vi "XYZStage-Request motor move all axes command.vi"(6 "Wait for acknowledge?":bool, 9 "Motor Z":sgl, 10 "Motor Y":sgl, 11 "Motor X":sgl) -> (1 "Timed out while waiting for acknowledgement":bool, 2 "Acknowledgement message":string)   [LabVIEW 2013]
doc: "Sends a request to the XYZ Stage driver to move the motor to the specified position on the Z axis."
uses:
  Typedefs/XYZ stage states.ctl
  Typedefs/XYZ stage data.ctl
  Typedefs/XYZ channel ring.ctl
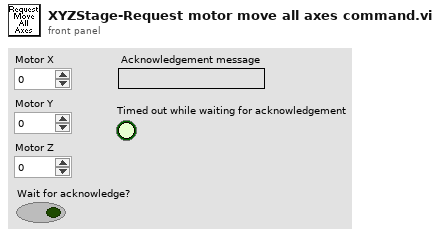
[diagram p1: front panel]
types:
  T1 = typedef "XYZ channel ring.ctl" = string
  T2 = typedef "XYZ stage data.ctl" = cluster{"Command":T3, "Channel":T1, "X":sgl, "Y":sgl, "Z":sgl, "Speed":i32, "Zero":bool, "Use acknowledgement?":bool}
  T3 = typedef "XYZ stage states.ctl" = enum16{"Dequeue", "Initialize", "Read Position", "Read Speed Setting", "Move", "Set Max Speed", "Reset Axis", "Stop all movement"}
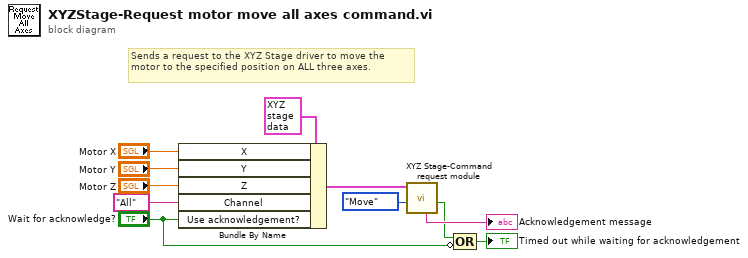
[diagram p0: block diagram]
diagram:
  # "Sends a request to the XYZ Stage driver to move the motor to the specified position on ALL three axes."
  n1 = Bundle By Name(cluster=T2 {"Command"=enum."Initialize", "Channel"="", "X"=0.0, "Y"=0.0, "Z"=0.0, "Speed"=0, "Zero"=TRUE, "Use acknowledgement?"=FALSE} ("XYZ Stage data to queue"), "X"="Motor X", "Y"="Motor Y", "Z"="Motor Z", "Channel"=T1 "All", "Use acknowledgement?"="Wait for acknowledge?") -> (w11:T2)
  n2 = call "XYZ Stage-Command request module.vi"("Command"=XYZ_stage_states."Move", "XYZ Stage data to queue"=w11) -> ("Timed out while waiting for acknowledgement"=w3:bool, "Acknowledgement message"=→"Acknowledgement message":string)  [unwired: 5 in, 3 out]
  n3 = Compound Arithmetic op=OR(w3, invert "Wait for acknowledge?") -> (→"Timed out while waiting for acknowledgement":bool)
